vi "Get Latest All.vi"(8 "error in (no error)":errorcluster, 11 "BME280 in":refnum<class "BME280.lvclass">) -> (0 "error out":errorcluster, 2 "Single Weather":T1, 3 "BME280 out":refnum<class "BME280.lvclass">)   [LabVIEW 2020, in "BME280.lvclass"]
uses:
  BME280.lvclass
  Single Weather.ctl
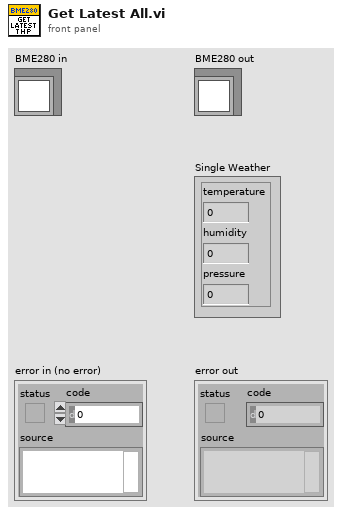
[diagram p1: front panel]
types:
  T1 = typedef "BME280.lvclass/Single Weather.ctl" = cluster{"temperature":dbl, "humidity":dbl, "pressure":dbl}
  T2 = typedef "BME280.lvclass/Weather.ctl" = cluster{"temperature":dbl[], "humidity":dbl[], "pressure":dbl[]}
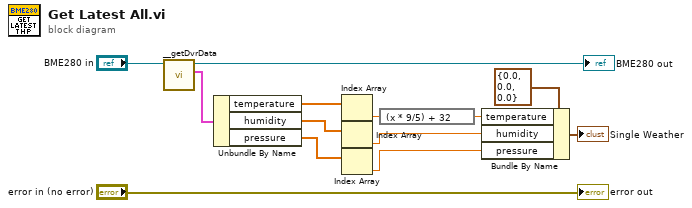
[diagram p0: block diagram]
diagram:
  n1 = call "__getDvrData.vi"("BME280 in"="BME280 in") -> ("weather"=w11:T2, "BME280 out"=→"BME280 out":refnum<class "BME280.lvclass">)  [unwired: 8 in, 1 out]
  n2 = Unbundle By Name(w11) -> ("temperature"=w10:dbl[], "humidity"=w9:dbl[], "pressure"=w8:dbl[])
  n3 = Index Array(array=w10) -> (element=w4:dbl)  [unwired: 1 in]
  n4 = Index Array(array=w9) -> (element=w2:dbl)  [unwired: 1 in]
  n5 = Index Array(array=w8) -> (element=w1:dbl)  [unwired: 1 in]
  n6 = expression code="(x * 9/5) + 32"(w4) -> (w3:dbl)
  n7 = Bundle By Name(cluster=T1 {"temperature"=0.0, "humidity"=0.0, "pressure"=0.0} ("singleWeather"), "temperature"=w3, "humidity"=w2, "pressure"=w1) -> (→"Single Weather":T1)
  "error out" <- "error in (no error)"
